vi "setOutputState.vi"(8 "error in (no error)":errorcluster, 9 "State":bool, 10 "Channel Nr (1)":string="1", 11 "VISA resource name":refnum<visa-resource-name>) -> (0 "error out":errorcluster, 3 "VISA resource name out":refnum<visa-resource-name>)   [LabVIEW 2023, in "Tti-Pl303Qmd.lvlib"]
doc: "Set Output State"
uses:
  Tti-Pl303Qmd.lvlib
  <vilib>/Utility/error.llb/Error Cluster From Error Code.vi
  <vilib>/ErrorRing/Error Ring.xnode
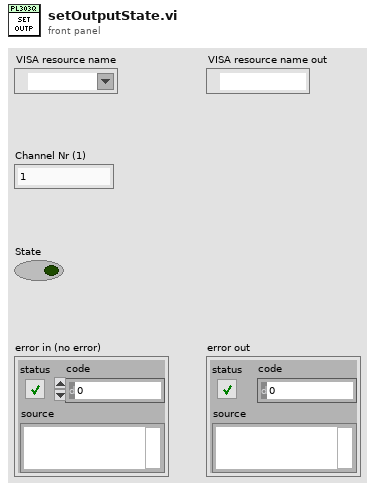
[diagram p1: front panel]
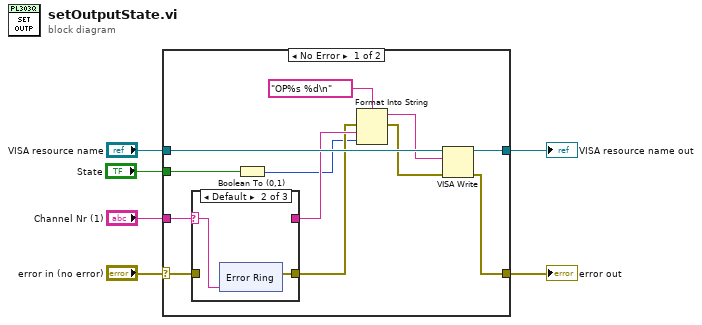
[diagram p0: block diagram]
diagram:
  n1 = case shown="No Error" "error in (no error)" {
    selector: "error in (no error)" -> [w15 w33]
    tunnel: "VISA resource name" -> [w17 w32]
    tunnel: [w18 w33] -> w6
    tunnel: "Channel Nr (1)" -> [w16 _]
    tunnel: [w9 w32] -> w2
    tunnel: "State" -> [w8 _]
    frame No Error {
      n2 = case shown="Default" w16 {
        selector: w16 -> [w20 w21 w30]
        tunnel: w15 -> [w19 _ w31]
        tunnel: [w19 w22 w31] -> w12
        tunnel: [w20 _ w30] -> w13
        frame "2" {
        }
        frame Default {
          n3 = xnode "Error Ring"("parameter 0"=w21) -> ("error out"=w22:errorcluster)
        }
        frame "1" {
        }
      }
      n4 = Boolean To (0,1)(Boolean=w8) -> (0, 1=w7:i16)
      n5 = Format Into String(format string="OP%s %d\n" ("write buffer"), error in=w12, w13, w7) -> (resulting string=w10:string, error out=w11:errorcluster)  [unwired: 1 in]
      n6 = VISA Write(VISA resource name=w17, write buffer=w10, error in (no error)=w11) -> (VISA resource name out=w9:refnum<visa-resource-name>, error out=w18:errorcluster)  [unwired: 1 out]
    }
    frame Error {
    }
  }
  "error out" <- w6
  "VISA resource name out" <- w2
